vi "ingresarDatosEquipos.vi"(8 "error in":errorcluster, 11 "Sonometro in":refnum<class "Sonometro.lvclass">) -> (0 "error out":errorcluster, 3 "Sonometro out":refnum<class "Sonometro.lvclass">)   [LabVIEW 2019, in "Sonometro.lvclass"]
uses:
  Sonometro.lvclass
  Sonometro.lvclass/Sonometro.ctl
  QMH/Message Queue/Enqueue Message (Single).vi
  <vilib>/Utility/error.llb/Error Cluster From Error Code.vi
  RerenceAllControlsToolkit/_get mutiple control reference by name.vi
  <vilib>/ErrorRing/Error Ring.xnode
  QMH/Message Queue/Message Queue.lvlib
  QMH/User Event - Stop/User Event - Stop.lvlib
panel:
  in  "Tab Control":enum32{"Datos de Equipos", "Datos de Cliente"}(tab)
  in  "guardar":bool
  in  "cb_marca_equipo":string(combo)
  in  "numero_serial_equipo":string
  in  "codigo_interno":string
  in  "cb_clase_equipo":string(combo)
  in  "cb_marca_mic":string(combo)
  in  "cb_marca_preamp":string(combo)
  in  "numero_serial_mic":string
  in  "cb_modelo_preamp":string(combo)
  in  "numero_serial_preamp":string
  in  "cb_modelo":string(combo)
  in  "cb_modelo_mic":string(combo)
  in  "salir":bool
  in  "DetalleCertificado":string[][](table)
  in  "Cliente":string[][](table)
  in  "DatosCertificado":string[][](table)=[[""], [""], [""], [""], [""], [""], [""]]
  out "Resultado":string
  # "Equipo"
  # "Micrófono"
  # "Preamplificador"
  # "Marca"
  # "Número de Serie"
  # "Código Interno"
  # "Clase"
  # "Marca"
  # "Modelo"
  # "Número Serial"
  # "Marca"
  # "Modelo"
  # "Número de Serie"
  # "Modelo"
  # "General Certificado de Calibración"
  # "Cliente"
  # "Detalles Certificado"
  # "Ingreso Datos de Instrumentos, Accesorios y Clientes"
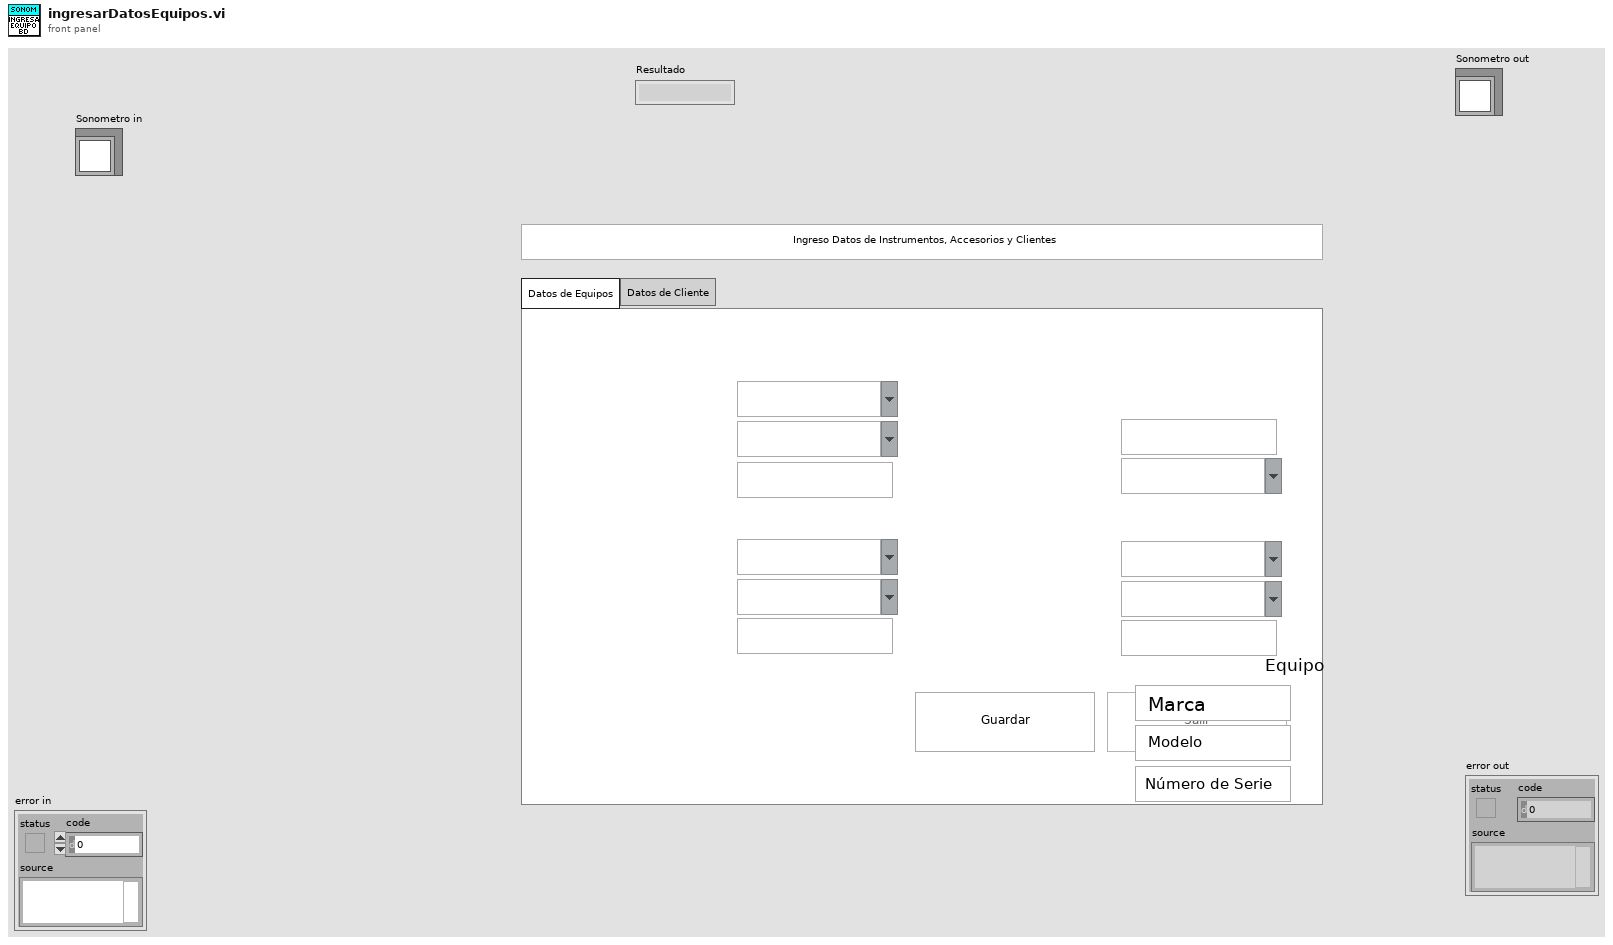
[diagram p1: front panel]
types:
  T1 = typedef "Message Queue.lvlib/All Message Queues.ctl" = cluster{"MHL":refnum<queue>, "Inst_CNT90":refnum<queue>, "Inst_DS360":refnum<queue>, "Inst_Keithley2002":refnum<queue>, "Inst_DAQ":refnum<queue>, "BD":refnum<queue>, "Pistofono":refnum<queue>, "Nexus":refnum<queue>}
  T2 = cluster{"ControlName":string, "ControlReference":refnum<vi>}[]
  T3 = cluster{string, "Control references":cluster{"ControlName":string, "ControlReference":refnum<vi>}[]}
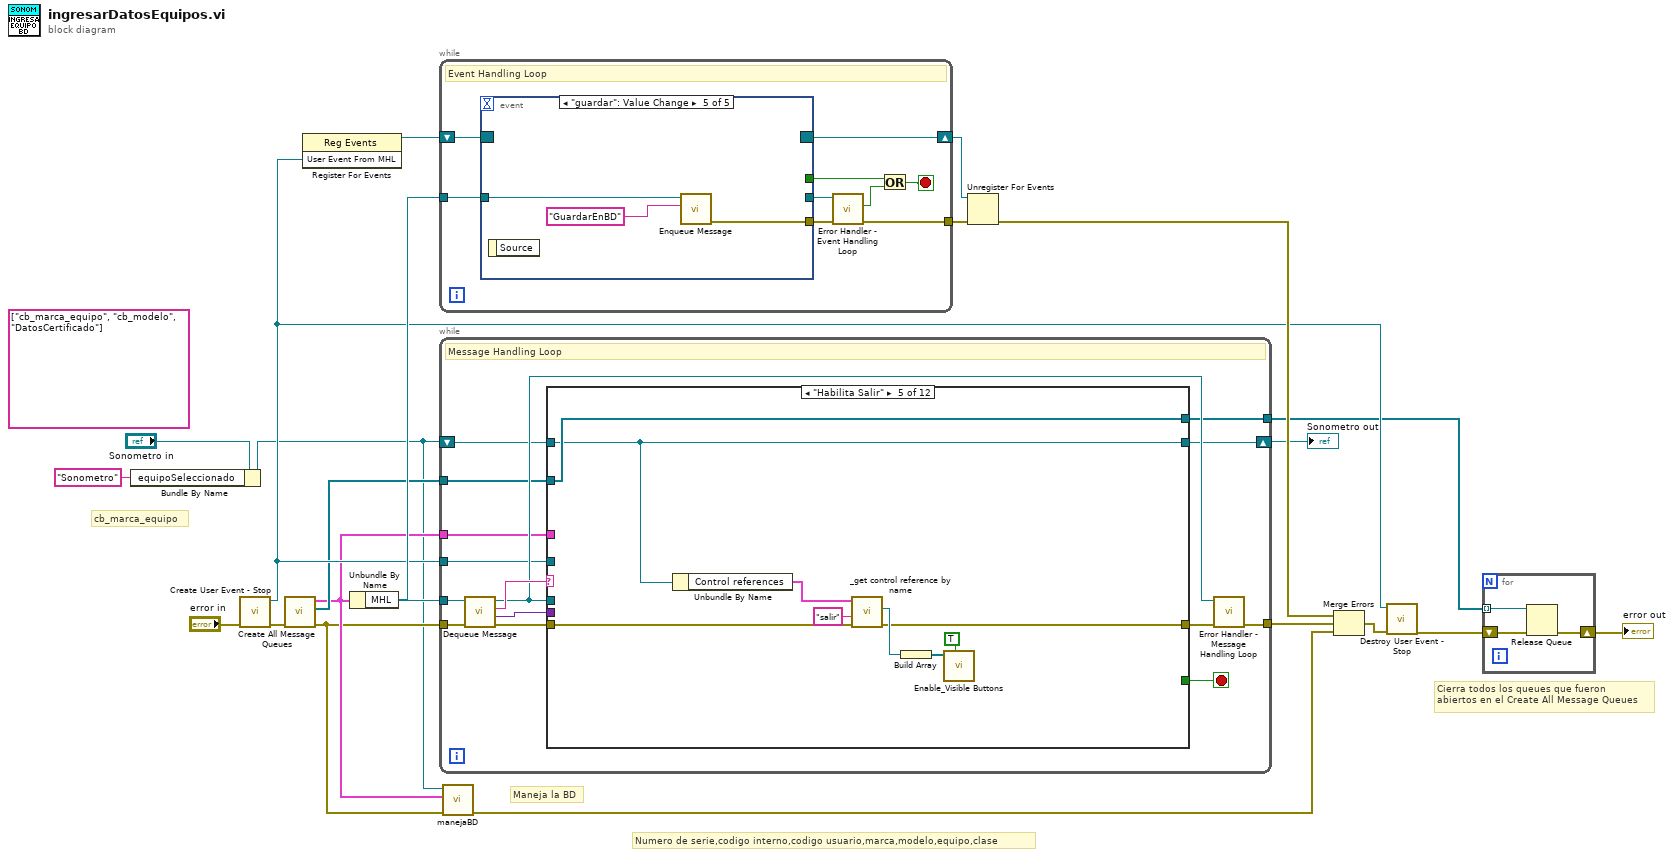
[diagram p0: block diagram]
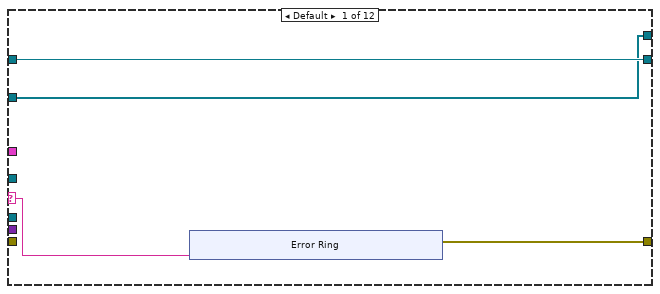
[diagram p2: hidden frame]
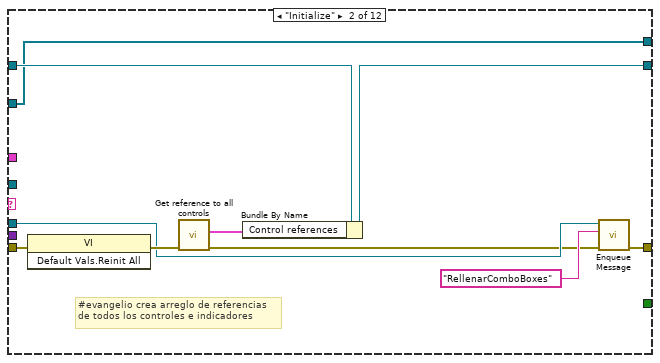
[diagram p3: hidden frame]
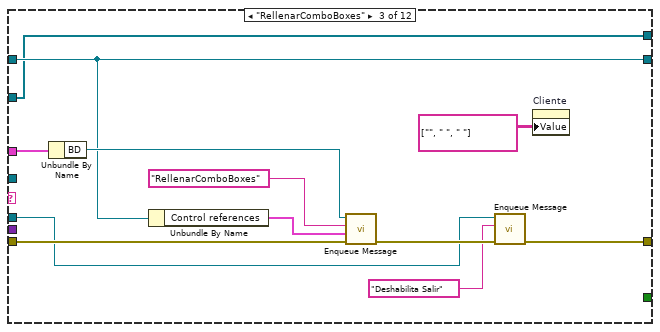
[diagram p4: hidden frame]
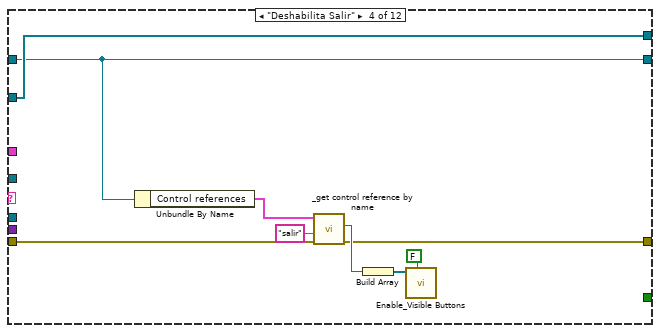
[diagram p5: hidden frame]
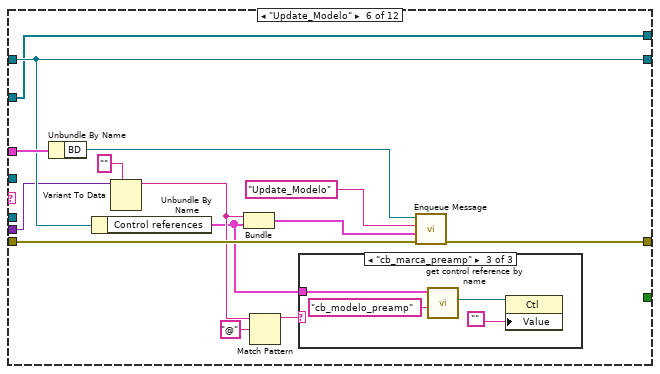
[diagram p6: hidden frame]
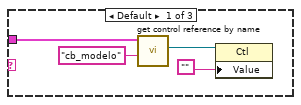
[diagram p7: hidden frame]
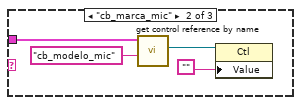
[diagram p8: hidden frame]
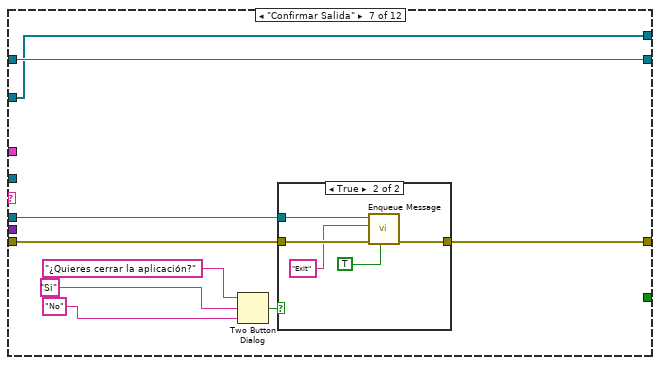
[diagram p9: hidden frame]
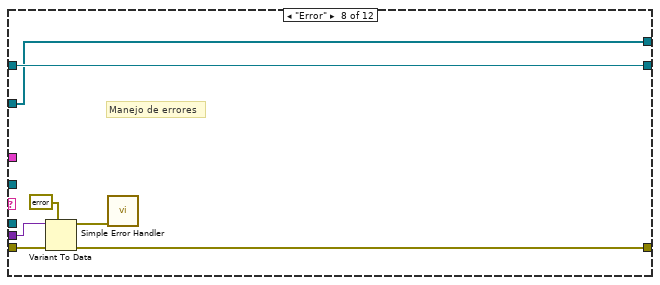
[diagram p11: hidden frame]
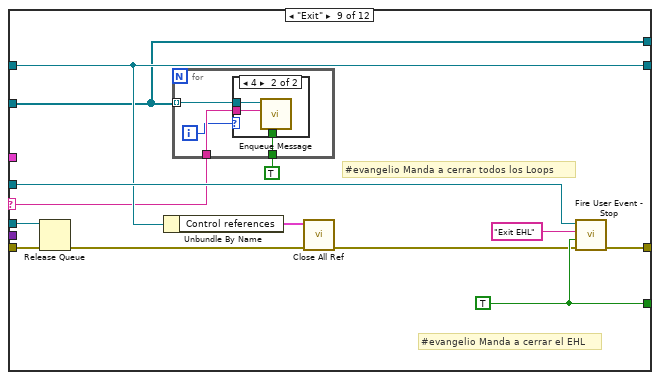
[diagram p12: hidden frame]
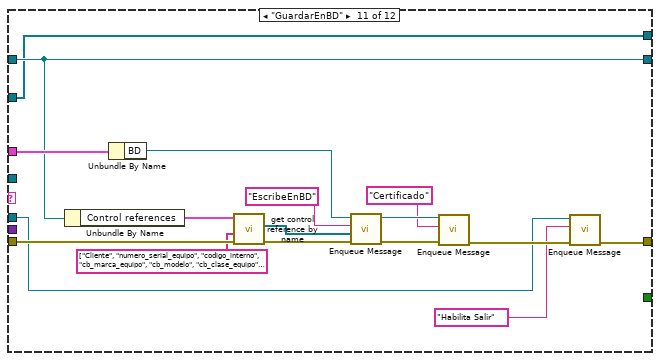
[diagram p15: hidden frame]
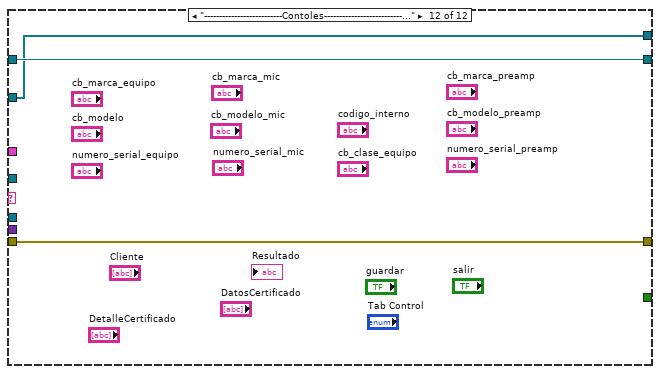
[diagram p16: hidden frame]
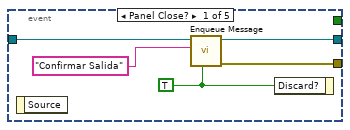
[diagram p17: hidden frame]
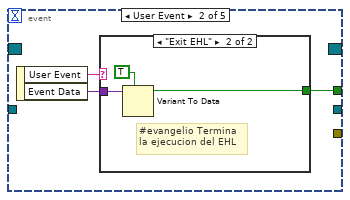
[diagram p18: hidden frame]
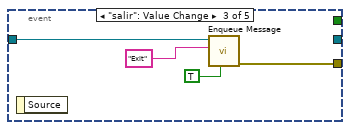
[diagram p20: hidden frame]
diagram:
  (unwired) string[] ["cb_marca_equipo", "cb_modelo", "DatosCertificado"]
  # "Cierra todos los queues que fueron\nabiertos en el Create All Message Queues"
  # "cb_marca_equipo"
  # "Numero de serie,codigo interno,codigo usuario,marca,modelo,equipo,clase"
  # "Maneja la BD"
  n1 = Bundle By Name(cluster="Sonometro in", "equipoSeleccionado"="Sonometro") -> (w5:refnum<class "Sonometro.lvclass">)
  n2 = call "Create User Event - Stop.vi"("error in (no error)"="error in") -> ("error out"=w18:errorcluster, "User Event From MHL"=w12:refnum<user-event>)  [unwired: 9 in]
  n3 = call "Create All Message Queues.vi"("error in (no error)"=w18) -> ("error out"=w8:errorcluster, "PL Queues Array"=w10:refnum<queue>[], "All Message Queues out"=w9:T1)  [unwired: 8 in]
  n4 = register-events(w12) -> (reference out=w21:refnum<event-registration>)  [unwired: 2 in, 1 out]
  n5 = Unbundle By Name(w9) -> ("MHL"=w17:refnum<queue>)
  n6 = while {
    tunnel: w17 -> [w30]
    tunnel: [w26] -> w20
    shift-right: [w28] -> w19
    shift-left: w21 -> [w29]
    stop <- w22 stop-if-true
    # "Event Handling Loop"
    n7 = event shown="[4] \"guardar\": Value Change" {
      selector: w29 -> [_ _ _ _ _]
      dyn-events: [_ _ _ _ _] -> w28
      timeout: _ -> [_ _ _ _ _]
      tunnel: w30 -> [w33 _ w44 w53 w56]
      tunnel: [w35 _ w45 w54 w57] -> w27
      tunnel: [w34 _ _ _ _] -> w25
      tunnel: [_ w36 _ _ _] -> w23
      event Panel Close? {
        w31 = TRUE
        n8 = event-data() -> ()  [unwired: 1 in, 1 out]
        n9 = call-poly "Enqueue Message.vi"("Priority Message? (F)"=w31, "Message"="Confirmar Salida", "Message Queue"=w33) -> ("error out"=w35:errorcluster, "dup Message Queue"=w34:refnum<queue>)  [unwired: 7 in]
        n10 = event-data("Discard?"=w31) -> ()  [unwired: 1 in, 1 out]
      }
      event User Event {
        n11 = event-data() -> ("User Event"=w38:string, "Event Data"=w37:variant)  [unwired: 1 in]
        n12 = case shown="\"Exit EHL\"" w38 {
          tunnel: w37 -> [_ w40]
          tunnel: [_ w39] -> w36
          frame Default {
          }
          frame "Exit EHL" {
            # "#evangelio Termina\nla ejecucion del EHL"
            n13 = Variant To Data(type=TRUE, Variant=w40) -> (data=w39:bool)  [unwired: 1 in, 1 out]
          }
        }
      }
      event "salir": Value Change {
        n14 = event-data() -> ()  [unwired: 1 in, 1 out]
        n15 = call-poly "Enqueue Message.vi"("Priority Message? (F)"=TRUE, "Message"="Exit", "Message Queue"=w44) -> ("error out"=w45:errorcluster)  [unwired: 7 in, 1 out]
      }
      event "cb_marca_equipo", "cb_marca_mic", "cb_marca_preamp": Value Change {
        n16 = event-data() -> ("CtlRef"=w50:refnum<vi>, "NewVal"=w49:string)  [unwired: 1 in]
        n17 = property class="CmbBox"(reference=w50) -> ("Label.Text"=w47:string)  [unwired: 1 in, 2 out]
        n18 = Concatenate Strings(w47, "@" ("string"), w49) -> (w48:string)
        n19 = call-poly "Enqueue Message.vi"("Priority Message? (F)"=TRUE, "Message Data"=w48, "Message"="Update_Modelo", "Message Queue"=w53) -> ("error out"=w54:errorcluster)  [unwired: 6 in, 1 out]
      }
      event "guardar": Value Change {
        n20 = event-data() -> ()  [unwired: 1 in, 1 out]
        n21 = call-poly "Enqueue Message.vi"("Message"="GuardarEnBD", "Message Queue"=w56) -> ("error out"=w57:errorcluster)  [unwired: 8 in, 1 out]
      }
    }
    n22 = call "Error Handler - Event Handling Loop.vi"("error in (no error)"=w27, "Message Queue"=w25) -> ("dup error in"=w26:errorcluster, "Error?"=w24:bool)  [unwired: 7 in, 1 out]
    n23 = Or(x=w23, y=w24) -> (x .or. y?=w22:bool)
  }
  n24 = while {
    tunnel: w8 -> [w72]
    tunnel: w17 -> [w71]
    tunnel: [w65] -> w15
    shift-right: [w63] -> w13
    shift-left: w5 -> [w64]
    tunnel: w9 -> [w61]
    tunnel: w12 -> [w60]
    tunnel: w10 -> [w59]
    tunnel: [w58] -> w2
    stop <- w62 stop-if-true
    # "Message Handling Loop"
    n25 = call "Dequeue Message.vi"("error in (no error)"=w72, "Message Queue"=w71) -> ("error out"=w68:errorcluster, "Message Data"=w69:variant, "Message"=w70:string, "dup Message Queue"=w67:refnum<queue>)  [unwired: 6 in]
    n26 = case shown="\"Habilita Salir\"" w70 {
      selector: w70 -> [w75 _ _ _ _ _ _ _ w175 _ _ _]
      tunnel: w67 -> [_ w90 w95 _ _ _ w151 _ w184 _ w196 _]
      tunnel: w69 -> [_ _ _ _ _ w131 _ w167 _ _ _ _]
      tunnel: w68 -> [_ w93 w105 w114 w123 w137 w157 w168 w183 w194 w208 w214]
      tunnel: [w74 w91 w96 w106 w115 w136 w156 w169 w182 w194 w197 w214] -> w66
      tunnel: w64 -> [w76 w86 w100 w112 w121 w132 w158 w171 w176 w193 w205 w213]
      tunnel: [w76 w88 w100 w112 w121 w132 w158 w171 w176 w193 w205 w213] -> w63
      tunnel: [_ _ _ _ _ _ _ _ w179 _ _ _] -> w62
      tunnel: w61 -> [_ _ w102 _ _ w134 _ _ _ _ w211 _]
      tunnel: w60 -> [_ _ _ _ _ _ _ _ w181 _ _ _]
      tunnel: w59 -> [w73 w84 w97 w113 w122 w124 w150 w165 w172 w192 w199 w212]
      tunnel: [w73 w84 w97 w113 w122 w124 w150 w165 w172 w192 w199 w212] -> w58
      frame Default {
        n27 = xnode "Error Ring"("parameter 0"=w75) -> ("error out"=w74:errorcluster)
      }
      frame "Initialize" {
        # "#evangelio crea arreglo de referencias\nde todos los controles e indicadores"
        n28 = invoke class="VI" method="Default Vals.Reinit All"(error in=w93) -> (error out=w92:errorcluster)  [unwired: 2 in, 2 out]
        n29 = call "Get reference to all controls.vi"("error in (no error)"=w92) -> ("error out"=w85:errorcluster, "Control references"=w87:T2)  [unwired: 5 in]
        n30 = Bundle By Name(cluster=w86, "Control references"=w87) -> (w88:refnum<class "Sonometro.lvclass">)
        n31 = call-poly "Enqueue Message.vi"("error in (no error)"=w85, "Message"="RellenarComboBoxes", "Message Queue"=w90) -> ("error out"=w91:errorcluster)  [unwired: 7 in, 1 out]
      }
      frame "RellenarComboBoxes" {
        n32 = Unbundle By Name(w102) -> ("BD"=w101:refnum<queue>)
        n33 = Unbundle By Name(w100) -> ("Control references"=w99:T2)
        n34 = call-poly "Enqueue Message.vi"("error in (no error)"=w105, "Message Data"=w99, "Message"="RellenarComboBoxes", "Message Queue"=w101) -> ("error out"=w104:errorcluster)  [unwired: 6 in, 1 out]
        n35 = call-poly "Enqueue Message.vi"("error in (no error)"=w104, "Message"="Deshabilita Salir", "Message Queue"=w95) -> ("error out"=w96:errorcluster)  [unwired: 7 in, 1 out]
        n36 = property on="Cliente" class="Tbl (strict)"("Value"=string[][] [[""], [" "], [" "]]) -> ()  [unwired: 2 in, 2 out]
      }
      frame "Deshabilita Salir" {
        n37 = Unbundle By Name(w112) -> ("Control references"=w111:T2)
        n38 = call "_get control reference by name.vi"("error in (no error)"=w114, "Control name"="salir", "Control references"=w111) -> ("error out"=w106:errorcluster, "Ctl Refnum"=w109:refnum<vi>)  [unwired: 3 in]
        n39 = Build Array(w109) -> (w108:refnum<vi>[])
        n40 = call "Enable_Visible Buttons.vi"("Enable? (T)"=FALSE, "Controls Ref Array"=w108) -> ()  [unwired: 10 in]
      }
      frame "Habilita Salir" {
        n41 = Unbundle By Name(w121) -> ("Control references"=w120:T2)
        n42 = call "_get control reference by name.vi"("error in (no error)"=w123, "Control name"="salir", "Control references"=w120) -> ("error out"=w115:errorcluster, "Ctl Refnum"=w118:refnum<vi>)  [unwired: 3 in]
        n43 = Build Array(w118) -> (w117:refnum<vi>[])
        n44 = call "Enable_Visible Buttons.vi"("Enable? (T)"=TRUE, "Controls Ref Array"=w117) -> ()  [unwired: 10 in]
      }
      frame "Update_Modelo" {
        n45 = Unbundle By Name(w134) -> ("BD"=w133:refnum<queue>)
        n46 = Unbundle By Name(w132) -> ("Control references"=w125:T2)
        n47 = Variant To Data(type="", Variant=w131) -> (data=w128:string)  [unwired: 1 in, 1 out]
        n48 = Bundle(w128, "Control references"=w125) -> (w129:T3)  [unwired: 1 in]
        n49 = Match Pattern(string=w128, regular expression="@") -> (before substring=w126:string)  [unwired: 1 in, 3 out]
        n50 = case shown="\"cb_marca_preamp\"" w126 {
          tunnel: w125 -> [w138 w142 w146]
          frame Default {
            n51 = call-poly "get control reference by name.vi"("Control name"="cb_modelo", "Control references"=w138) -> ("Ctl Refnum"=w139:refnum<vi>)  [unwired: 4 in, 1 out]
            n52 = property class="Ctl"(reference=w139, "Value"="") -> ()  [unwired: 1 in, 2 out]
          }
          frame "cb_marca_mic" {
            n53 = call-poly "get control reference by name.vi"("Control name"="cb_modelo_mic", "Control references"=w142) -> ("Ctl Refnum"=w143:refnum<vi>)  [unwired: 4 in, 1 out]
            n54 = property class="Ctl"(reference=w143, "Value"="") -> ()  [unwired: 1 in, 2 out]
          }
          frame "cb_marca_preamp" {
            n55 = call-poly "get control reference by name.vi"("Control name"="cb_modelo_preamp", "Control references"=w146) -> ("Ctl Refnum"=w147:refnum<vi>)  [unwired: 4 in, 1 out]
            n56 = property class="Ctl"(reference=w147, "Value"="") -> ()  [unwired: 1 in, 2 out]
          }
        }
        n57 = call-poly "Enqueue Message.vi"("error in (no error)"=w137, "Message Data"=w129, "Message"="Update_Modelo", "Message Queue"=w133) -> ("error out"=w136:errorcluster)  [unwired: 6 in, 1 out]
      }
      frame "Confirmar Salida" {
        n58 = Two Button Dialog(message="¿Quieres cerrar la aplicación?", 1:"No" ("T button name (\"OK\")"), 2:"Si" ("T button name (\"OK\")")) -> (T button?=w152:bool)
        n59 = case shown="True" w152 {
          tunnel: w157 -> [w159 w164]
          tunnel: [w159 w163] -> w156
          tunnel: w151 -> [_ w162]
          frame False {
          }
          frame True {
            n60 = call-poly "Enqueue Message.vi"("Priority Message? (F)"=TRUE, "error in (no error)"=w164, "Message"="Exit", "Message Queue"=w162) -> ("error out"=w163:errorcluster)  [unwired: 6 in, 1 out]
          }
        }
      }
      frame "Error" {
        # "Manejo de errores"
        n61 = Variant To Data(error in=w168, type=errorcluster {"status"=FALSE, "code"=0, "source"=""} ("error constant"), Variant=w167) -> (data=w166:errorcluster, error out=w169:errorcluster)
        n62 = call <vilib>:"Simple Error Handler.vi"("error in (no error)"=w166) -> ()  [unwired: 4 in, 5 out]
      }
      frame "Exit" {
        w179 = TRUE
        # "#evangelio Manda a cerrar todos los Loops"
        # "#evangelio Manda a cerrar el EHL"
        n63 = Release Queue(queue=w184, error in (no error)=w183) -> (error out=w174:errorcluster)  [unwired: 1 in, 2 out]
        n64 = Unbundle By Name(w176) -> ("Control references"=w178:T2)
        n65 = for {
          tunnel: w172 -> [w188] mode=indexing
          tunnel: w175 -> [w187]
          tunnel: TRUE -> [w186]
          i -> [w185]
          n66 = case shown="4" w185 {
            tunnel: w188 -> [_ w191]
            tunnel: w187 -> [_ w190]
            tunnel: w186 -> [_ w189]
            frame Default {
            }
            frame 4 {
              n67 = call-poly "Enqueue Message.vi"("Priority Message? (F)"=w189, "Message"=w190, "Message Queue"=w191) -> ()  [unwired: 7 in, 2 out]
            }
          }
        }
        n68 = call "Close All Ref.vi"("error in (no error)"=w174, "Control references"=w178) -> ("error out"=w173:errorcluster)  [unwired: 9 in]
        n69 = call "Fire User Event - Stop.vi"("error in (no error)"=w173, "Event Data"=w179, "User Event"="Exit EHL", "User Event in"=w181) -> ("error out"=w182:errorcluster)  [unwired: 7 in]
      }
      frame "---- BD ----" {
      }
      frame "GuardarEnBD" {
        n70 = Unbundle By Name(w205) -> ("Control references"=w206:T2)
        n71 = Unbundle By Name(w211) -> ("BD"=w210:refnum<queue>)
        n72 = call-poly "get control reference by name.vi"("error in (no error)"=w208, "Control names"=string[] ["Cliente", "numero_serial_equipo", "codigo_interno", "cb_marca_equipo", "cb_modelo", "cb_clase_equipo", "cb_marca_mic", "cb_modelo_mic", "numero_serial_mic", "cb_marca_preamp", "cb_modelo_preamp", "numero_serial_preamp"], "Control references"=w206) -> ("error out"=w207:errorcluster, "References"=w200:refnum<vi>[])  [unwired: 3 in]
        n73 = call-poly "Enqueue Message.vi"("error in (no error)"=w207, "Message Data"=w200, "Message"="EscribeEnBD", "Message Queue"=w210) -> ("error out"=w203:errorcluster, "dup Message Queue"=w202:refnum<queue>)  [unwired: 6 in]
        n74 = call-poly "Enqueue Message.vi"("error in (no error)"=w203, "Message"="Certificado", "Message Queue"=w202) -> ("error out"=w198:errorcluster)  [unwired: 7 in, 1 out]
        n75 = call-poly "Enqueue Message.vi"("error in (no error)"=w198, "Message"="Habilita Salir", "Message Queue"=w196) -> ("error out"=w197:errorcluster)  [unwired: 7 in, 1 out]
      }
      frame "--------------------------Contoles---------------------------" {
      }
    }
    n76 = call "Error Handler - Message Handling Loop.vi"("error in (no error)"=w66, "Message Queue"=w67) -> ("dup error in"=w65:errorcluster)  [unwired: 8 in, 1 out]
  }
  "Sonometro out" <- w13
  n77 = call "manejaBD.vi"("error in"=w8, "All Message Queues in"=w9, "Sonometro in"=w5) -> ("error out"=w1:errorcluster)  [unwired: 8 in]
  n78 = Unregister For Events(event registration refnum=w19, error in=w20) -> (error out=w16:errorcluster)
  n79 = Merge Errors(w16, w15, w1) -> (w14:errorcluster)
  n80 = call "Destroy User Event - Stop.vi"("error in (no error)"=w14, "User Event"=w12) -> ("error out"=w4:errorcluster)  [unwired: 9 in]
  n81 = for {
    shift-right: [w216] -> w3
    shift-left: w4 -> [w217]
    tunnel: w2 -> [w215] mode=indexing
    n82 = Release Queue(queue=w215, error in (no error)=w217) -> (error out=w216:errorcluster)  [unwired: 1 in, 2 out]
  }
  "error out" <- w3
